vi "Create.vi"(8 "error in (no error)":errorcluster) -> (0 "error out":errorcluster, 3 "QR Code Detector":refnum<class "QR Code Detector.lvclass">)   [LabVIEW 2020, in "feature_detection.lvlib" / "QR Code Detector.lvclass"]
doc: "Create a QR Code detector. This detector generally performs worse than the WeChat QR Code detector but provides a more flexible API for different tasks associated with QR Code detection and supports \"Structured Append\" mode QR Codes."
uses:
  QR Code Detector.lvclass
  QR Code Detector.lvclass/QR Code Detector.ctl
  common/common.lvlib
  common/bin/gartoolkit_32-1.dll
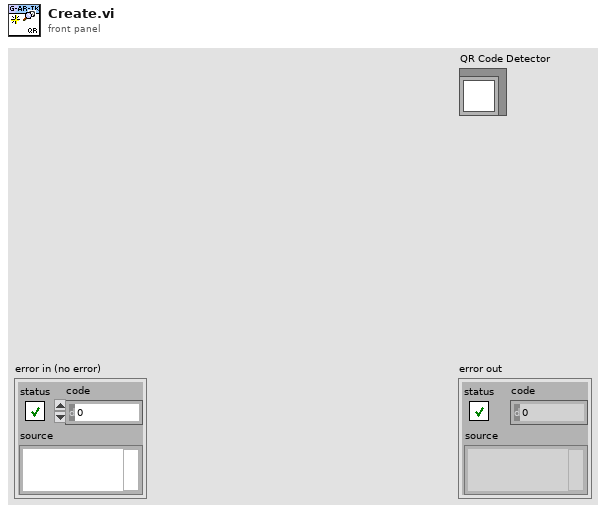
[diagram p1: front panel]
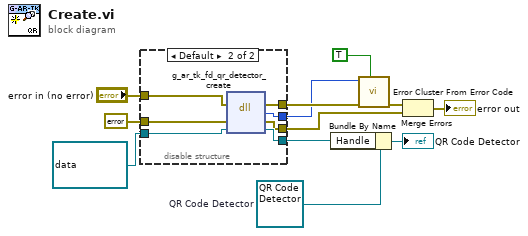
[diagram p0: block diagram]
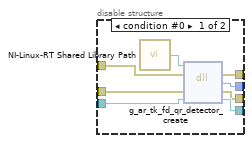
[diagram p2: hidden frame]
diagram:
  w12 = refnum<class "QR Code Detector.lvclass"> refnum  # QR Code Detector
  n1 = disable-structure "Conditional Disable Structure" shown="Default" {
    disable-tunnel: "error in (no error)" -> [w20 w27]
    disable-tunnel: errorcluster {"status"=FALSE, "code"=0, "source"=""} ("error constant") -> [w16 w26]
    disable-tunnel: refnum<data-value> refnum ("EDVR") -> [w15 w25]
    disable-tunnel: [w19 w24] -> w6
    disable-tunnel: [w18 w23] -> w5
    disable-tunnel: [w14 w22] -> w4
    disable-tunnel: [w13 w21] -> w2
    frame condition #0 {
      n2 = call "NI-Linux-RT Shared Library Path.vi"() -> ("Path"=w17:path)
      n3 = dll-call lib="?" fn="g_ar_tk_fd_qr_detector_create" ("g_ar_toolkit.*.*:g_ar_tk_capture_context_create")(path in=w17, error in=w20, "error_cluster"=w16, "EDVR"=w15) -> (error out=w19:errorcluster, w18:i32, "error_cluster"=w13:errorcluster, "EDVR"=w14:refnum<data-value>)  [unwired: 1 in, 1 out]
    }
    frame condition #1 (active) {
      n4 = dll-call lib="C:/Workspace/CSS/g-augmented-reality-toolkit/LabVIEW/common/bin/gartoolkit_*-1.*" fn="g_ar_tk_fd_qr_detector_create" ("g_ar_toolkit.*.*:g_ar_tk_capture_context_create")(error in=w27, "error_cluster"=w26, "EDVR"=w25) -> (error out=w24:errorcluster, "return type"=w23:i32, "error_cluster"=w21:errorcluster, "EDVR"=w22:refnum<data-value>)  [unwired: 2 in, 1 out]
    }
  }
  n5 = Bundle By Name(cluster=w12, "Handle"=w4) -> (→"QR Code Detector":refnum<class "QR Code Detector.lvclass">)
  n6 = call <vilib>:"Error Cluster From Error Code.vi"("show call chain? (False)"=TRUE, "error in (no error)"=w6, "error code (0)"=w5) -> ("error out"=w10:errorcluster)  [unwired: 6 in]
  n7 = Merge Errors(w10, w2) -> (→"error out":errorcluster)
